vi "MT Generate CPM Synchronization Parameters (bit array).vi"(0 "CPM system parameters":T1={"samples per symbol (16)"=16, "symbol map"=[]}, 5 "sync bits":i8[](array[numeric]), 11 "error in (no error)":errorcluster, 12 "expected sync location (symbols)":i32=-1, 13 "sync location uncertainty (symbols)":i32=10, 14 "sync indent (symbols)":i32) -> (4 "CPM synchronization parameters":T2 {"sync sequence" format="%.2f"}, 15 "error out":errorcluster)   [LabVIEW 2020, in "niDMT.lvlib"]
doc: "This polymorphic instance generates synchronization parameters for CPM demodulation using a synchronization sequence directly represented by the <B>sync bits</B> array."
uses:
  <vilib>/addons/Modulation/niDMT.lvlib
  <vilib>/addons/Modulation/Digital/Support/Controls/CPM System Parameters.ctl
  <vilib>/addons/Modulation/niAMT.lvlib
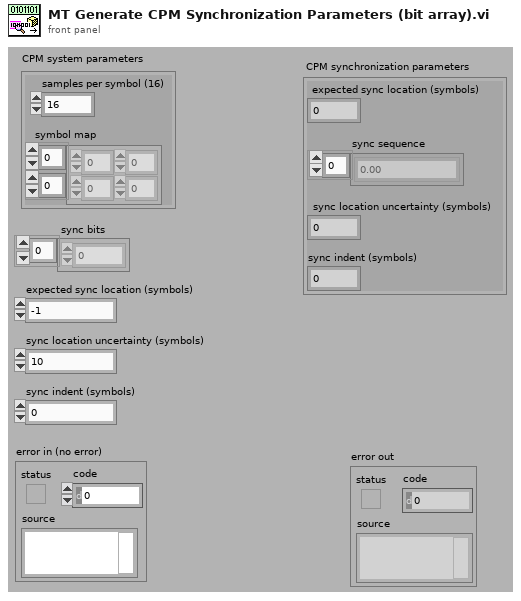
[diagram p1: front panel]
types:
  T1 = typedef "niDMT.lvlib/CPM System Parameters.ctl" = cluster{"samples per symbol (16)":i32, "symbol map":dbl[][]}
  T2 = cluster{"expected sync location (symbols)":i32, "sync sequence":cdb[], "sync location uncertainty (symbols)":i32, "sync indent (symbols)":i32}
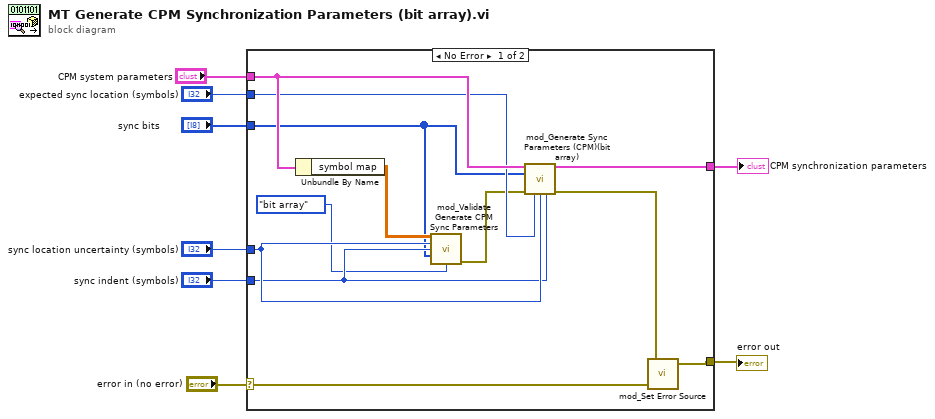
[diagram p0: block diagram]
diagram:
  n1 = case shown="No Error" "error in (no error)" {
    selector: "error in (no error)" -> [w19 w21]
    tunnel: "CPM system parameters" -> [w17 _]
    tunnel: "expected sync location (symbols)" -> [w15 _]
    tunnel: "sync location uncertainty (symbols)" -> [w13 _]
    tunnel: "sync indent (symbols)" -> [w12 _]
    tunnel: "sync bits" -> [w11 _]
    tunnel: [w20 w21] -> w2
    tunnel: [w16 _] -> w1
    frame No Error {
      n2 = Unbundle By Name(w17) -> ("symbol map"=w14:dbl[][])
      n3 = call <vilib>:"mod_Validate Generate CPM Sync Parameters.vi"("symbol map"=w14, "sync location uncertainty (symbols)"=w13, "sync indent (symbols)"=w12, "sync bits"=w11, "sync bits specification"=enum16{"bit array", "number array", "number"}."bit array") -> ("error out"=w9:errorcluster)  [unwired: 2 in, 8 out]
      n4 = call <vilib>:"mod_Generate Sync Parameters (CPM)(bit array).vi"("CPM system parameters"=w17, "sync bits"=w11, "error in (no error)"=w9, "expected sync location (symbols)"=w15, "sync location uncertainty (symbols)"=w13, "sync indent (symbols)"=w12) -> ("CPM synchronization parameters"=w16:T2, "error out"=w18:errorcluster)  [unwired: 8 out]
      n5 = call <vilib>:"mod_Set Error Source.vi"("initial error in (no error)"=w19, "final error in (no error)"=w18) -> ("error out"=w20:errorcluster)  [unwired: 3 out]
    }
    frame Error {
    }
  }
  "CPM synchronization parameters" <- w1
  "error out" <- w2
